vi "StartCore.vi"(8 "error in (no error)":errorcluster, 9 "Simulate?":bool, 10 "Service Details In":T1, 11 "MicronClient in":refnum<class "MicronClient.lvclass">) -> (0 "error out":errorcluster, 1 "Service Details Out":T1, 2 "Connection String":string, 3 "MicronClient out":refnum<class "MicronClient.lvclass">)   [LabVIEW 2019, in "MicronClient.lvclass"]
uses:
  MicronClient.lvclass
  Typedefs/ServiceDetails.ctl
  MicronCLI/Typedefs/Message.ctl
  MicronCLI/Typedefs/ServiceDetails.ctl
  824b107a-0fc2-4113-b1bd-0776a5adb667.vi
  <vilib>/SLL Toolkit/SLL String/_SubVIs/1D String Array to String.vi
  MicronCLI/MicronCLI.lvclass
  <vilib>/SLL Toolkit/SLL String/SLL String.lvlib
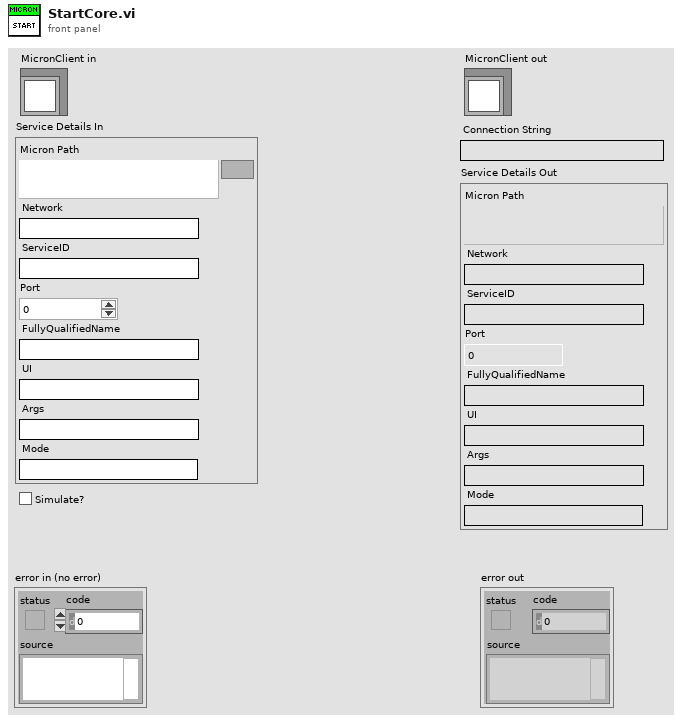
[diagram p1: front panel]
types:
  T1 = typedef "MicronClient.lvclass/ServiceDetails.ctl" = cluster{"Micron Path":path, "Network":string, "ServiceID":string, "Port":i32, "FullyQualifiedName":string, "UI":string, "Args":string, "Mode":string}
  T2 = typedef "MicronCLI.lvclass/Message.ctl" = cluster{"Command":string, "Payload":string}
  T3 = typedef "MicronCLI.lvclass/ServiceDetails.ctl" = cluster{"Network":string, "ServiceID":string}
  T4 = typedef "MicronClient.lvclass/MicronModeINISection.ctl" = cluster{"Command":string, "WorkingDirectory":path}
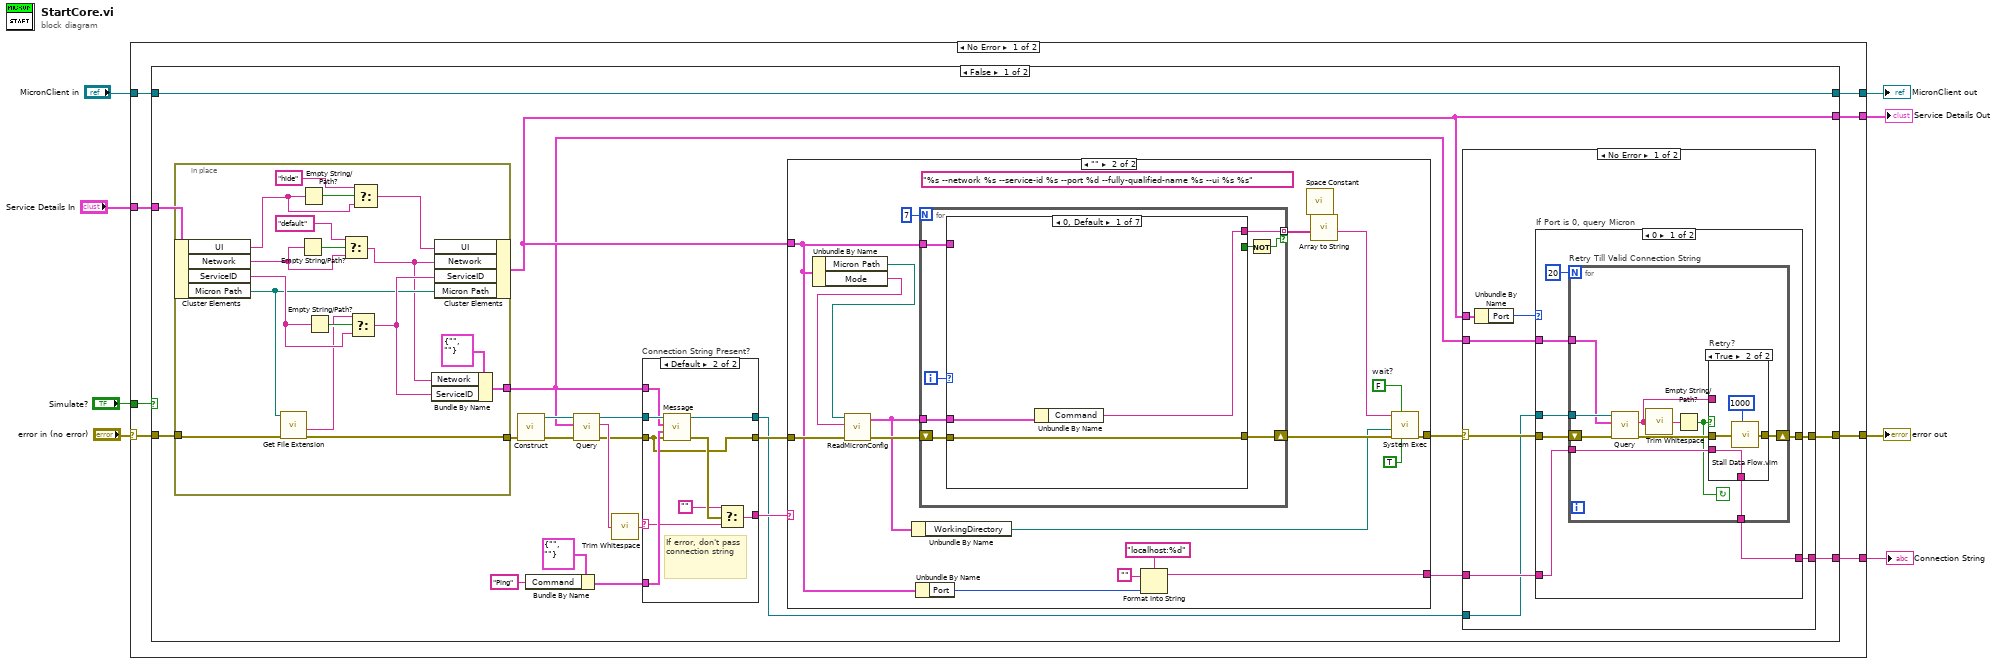
[diagram p0: block diagram]
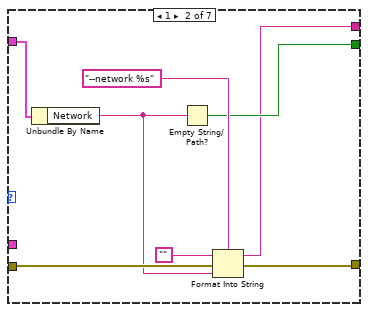
[diagram p7: hidden frame]
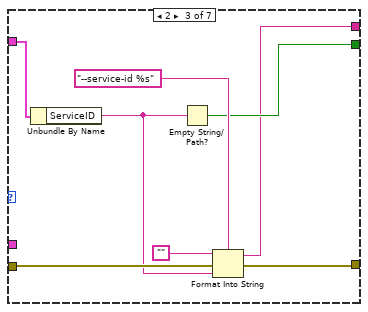
[diagram p8: hidden frame]
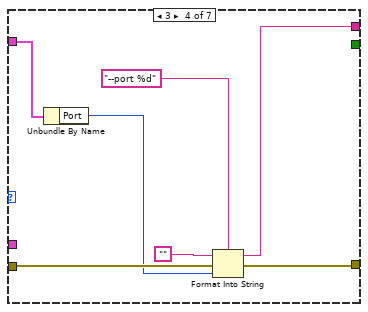
[diagram p9: hidden frame]
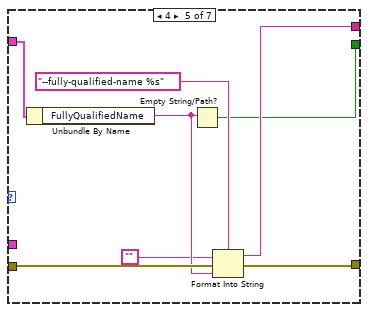
[diagram p10: hidden frame]
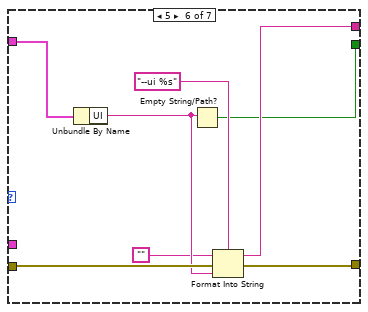
[diagram p11: hidden frame]
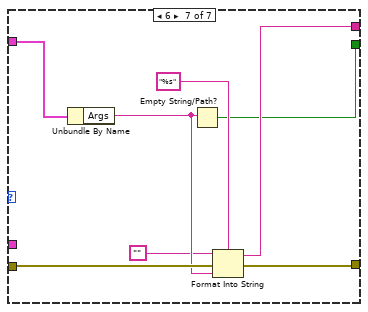
[diagram p12: hidden frame]
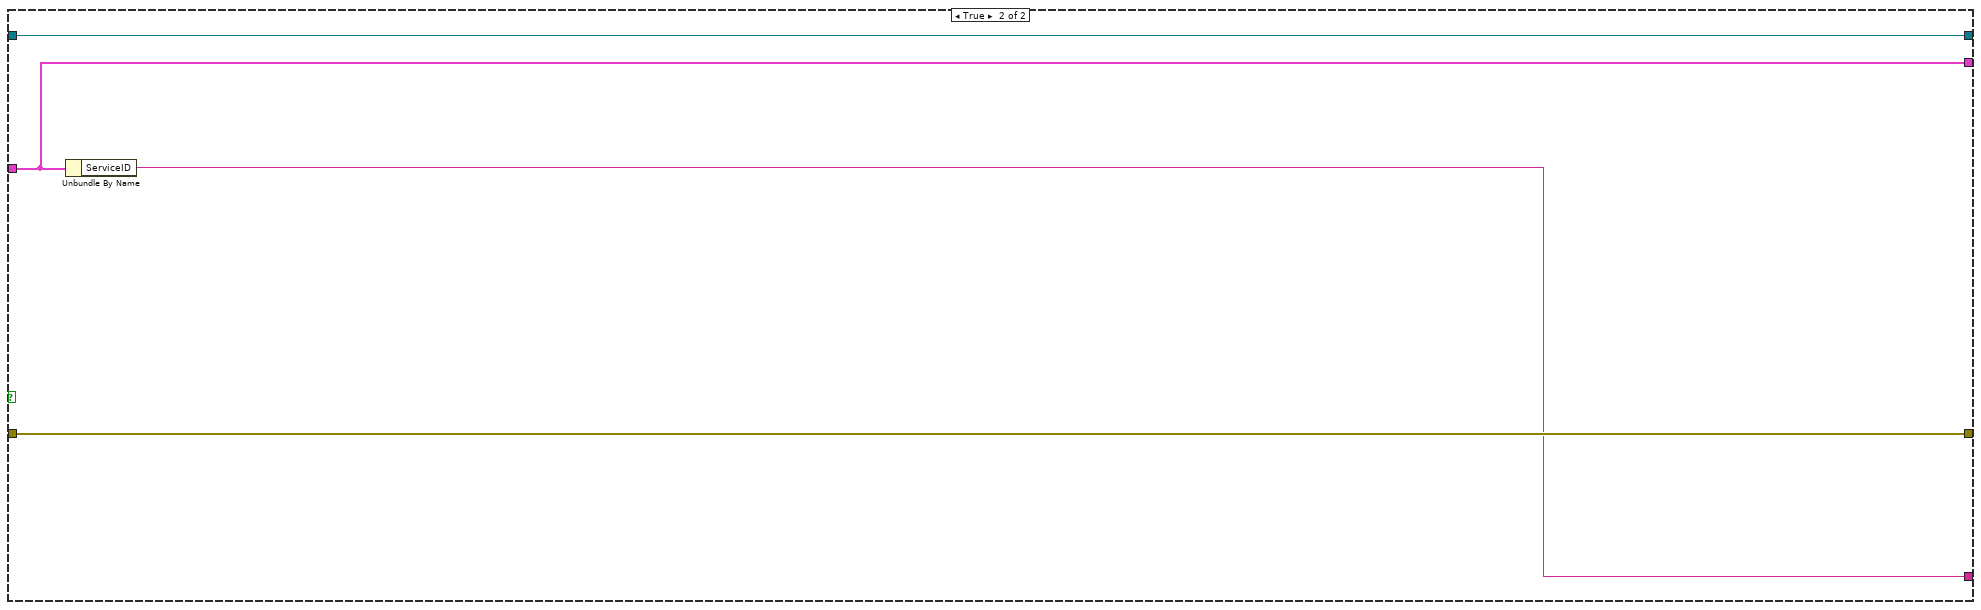
[diagram p13: hidden frame]
diagram:
  n1 = case shown="No Error" "error in (no error)" {
    selector: "error in (no error)" -> [w14 w188]
    tunnel: [w16 w188] -> w7
    tunnel: [w11 w187] -> w5
    tunnel: "MicronClient in" -> [w10 w187]
    tunnel: [w13 _] -> w4
    tunnel: "Service Details In" -> [w15 w186]
    tunnel: "Simulate?" -> [w12 _]
    tunnel: [w9 w186] -> w1
    frame No Error {
      n2 = case shown="False" w12 {
        tunnel: [w27 w185] -> w16
        tunnel: w15 -> [w38 w182]
        tunnel: w14 -> [w37 w185]
        tunnel: [w28 w183] -> w13
        tunnel: [w34 w184] -> w11
        tunnel: w10 -> [w34 w184]
        tunnel: [w30 w182] -> w9
        frame False {
          n3 = in-place {
            in-place-border: w37 -> [w178]
            in-place-border: [w174] -> w36
            in-place-border: [w165] -> w17
            n4 = in-place-cluster #1(w38) -> ("UI"=w170:string, "Network"=w180:string, "ServiceID"=w176:string, "Micron Path"=w173:path)
            n5 = call <vilib>:"Get File Extension.vi"("error in (no error)"=w178, "file"=w173) -> ("error out"=w174:errorcluster, "filename without extension"=w172:string)  [unwired: 5 in, 3 out]
            n6 = Empty String/Path?(string/path=w180) -> (empty?=w181:bool)
            n7 = Empty String/Path?(string/path=w170) -> (empty?=w171:bool)
            n8 = Empty String/Path?(string/path=w176) -> (empty?=w177:bool)
            n9 = Select(t="default", s=w181, f=w180) -> (s? t:f=w167:string)
            n10 = Select(t=w172, s=w177, f=w176) -> (s? t:f=w175:string)
            n11 = Select(t="hide", s=w171, f=w170) -> (s? t:f=w168:string)
            n12 = Bundle By Name(cluster=T3 {"Network"="", "ServiceID"=""} ("Service"), "Network"=w167, "ServiceID"=w175) -> (w165:T3)
            n13 = in-place-cluster #1("UI"=w168, "Network"=w167, "ServiceID"=w175, "Micron Path"=w173) -> (w30:T1)
          }
          n14 = call "Construct.vi"("error in (no error)"=w36) -> ("error out"=w33:errorcluster, "MicronCLI out"=w32:refnum<class "MicronCLI.lvclass">)  [unwired: 9 in]
          n15 = Bundle By Name(cluster=T2 {"Command"="", "Payload"=""} ("Message"), "Command"="Ping") -> (w18:T2)
          n16 = call-dynamic "Query.vi"("error in (no error)"=w33, "Service"=w17, "MicronCLI in"=w32) -> ("error out"=w26:errorcluster, "ConnectionString"=w35:string, "MicronCLI out"=w25:refnum<class "MicronCLI.lvclass">)  [unwired: 6 in]
          n17 = call <vilib>:"Trim Whitespace.vi"("string"=w35) -> ("trimmed string"=w24:string)  [unwired: 1 in]
          n18 = case "Connection String Present?" shown="Default" w24 {
            selector: w24 -> [w75 w79]
            tunnel: w26 -> [w76 w77]
            tunnel: w25 -> [w74 w85]
            tunnel: w17 -> [_ w84]
            tunnel: [w76 w77] -> w23
            tunnel: [w75 w78] -> w22
            tunnel: [w74 w83] -> w21
            tunnel: w18 -> [_ w82]
            frame "" {
            }
            frame Default {
              # "If error, don't pass connection string"
              n19 = call-dynamic "Message.vi"("error in (no error)"=w77, "Message"=w82, "Service"=w84, "MicronCLI in"=w85) -> ("error out"=w81:errorcluster, "MicronCLI out"=w83:refnum<class "MicronCLI.lvclass">)  [unwired: 5 in, 1 out]
              n20 = Select(t="", s=w81, f=w79) -> (s? t:f=w78:string)
            }
          }
          n21 = case shown="\"\"" w22 {
            selector: w22 -> [w87 _]
            tunnel: [w86 w98] -> w29
            tunnel: w30 -> [_ w92]
            tunnel: [w87 w96] -> w31
            tunnel: w23 -> [w86 w94]
            frame Default {
            }
            frame "" {
              (unwired) "%s --network %s --service-id %s --port %d --fully-qualified-name %s --ui %s %s" ("format string")
              w106 = FALSE  # wait?
              n22 = Unbundle By Name(w92) -> ("Micron Path"=w91:path, "Mode"=w88:string)
              n23 = call "ReadMicronConfig.vi"("Error In"=w94, "Mode"=w88, "Micron Path In"=w91) -> ("Error Out"=w93:errorcluster, "Micron Mode"=w90:T4)  [unwired: 7 in]
              n24 = Unbundle By Name(w90) -> ("WorkingDirectory"=w89:path)
              n25 = Unbundle By Name(w92) -> ("Port"=w97:i32)
              n26 = for {
                N: 7 -> [_]
                tunnel: w92 -> [w113]
                shift-right: [w111] -> w105
                shift-left: w93 -> [w112]
                tunnel: [w110] -> w101 mode=indexing if=w108
                tunnel: w90 -> [w107]
                i -> [w114]
                n27 = case shown="0, Default" w114 {
                  tunnel: w113 -> [_ w125 w133 w140 w148 w156 w164]
                  tunnel: w112 -> [w115 w124 w132 w139 w147 w155 w163]
                  tunnel: [w115 w123 w131 w138 w146 w154 w162] -> w111
                  tunnel: [w117 w119 w127 w135 w144 w152 w160] -> w110
                  tunnel: [_ w120 w128 _ w142 w150 w158] -> w109
                  tunnel: w107 -> [w116 _ _ _ _ _ _]
                  frame 0, Default {
                    n28 = Unbundle By Name(w116) -> ("Command"=w117:string)
                  }
                  frame 1 {
                    n29 = Unbundle By Name(w125) -> ("Network"=w121:string)
                    n30 = Empty String/Path?(string/path=w121) -> (empty?=w120:bool)
                    n31 = Format Into String(format string="--network %s", initial string="", error in=w124, w121) -> (resulting string=w119:string, error out=w123:errorcluster)
                  }
                  frame 2 {
                    n32 = Unbundle By Name(w133) -> ("ServiceID"=w129:string)
                    n33 = Empty String/Path?(string/path=w129) -> (empty?=w128:bool)
                    n34 = Format Into String(format string="--service-id %s", initial string="", error in=w132, w129) -> (resulting string=w127:string, error out=w131:errorcluster)
                  }
                  frame 3 {
                    n35 = Unbundle By Name(w140) -> ("Port"=w136:i32)
                    n36 = Format Into String(format string="--port %d", initial string="", error in=w139, w136) -> (resulting string=w135:string, error out=w138:errorcluster)
                  }
                  frame 4 {
                    n37 = Unbundle By Name(w148) -> ("FullyQualifiedName"=w143:string)
                    n38 = Empty String/Path?(string/path=w143) -> (empty?=w142:bool)
                    n39 = Format Into String(format string="--fully-qualified-name %s", initial string="", error in=w147, w143) -> (resulting string=w144:string, error out=w146:errorcluster)
                  }
                  frame 5 {
                    n40 = Unbundle By Name(w156) -> ("UI"=w151:string)
                    n41 = Empty String/Path?(string/path=w151) -> (empty?=w150:bool)
                    n42 = Format Into String(format string="--ui %s", initial string="", error in=w155, w151) -> (resulting string=w152:string, error out=w154:errorcluster)
                  }
                  frame 6 {
                    n43 = Unbundle By Name(w164) -> ("Args"=w159:string)
                    n44 = Empty String/Path?(string/path=w159) -> (empty?=w158:bool)
                    n45 = Format Into String(format string="%s", initial string="", error in=w163, w159) -> (resulting string=w160:string, error out=w162:errorcluster)
                  }
                }
                n46 = Not(x=w109) -> (.not. x?=w108:bool)
              }
              n47 = Format Into String(format string="localhost:%d", initial string="", w97) -> (resulting string=w96:string)  [unwired: 1 in, 1 out]
              n48 = call <vilib>:"Space Constant.vi"() -> ("String"=w100:string)
              n49 = call-poly <vilib>:"Array to String.vi"("Delimiter (,)"=w100, "1D Array[]"=w101) -> ("String"=w104:string)  [unwired: 6 in]
              n50 = call <vilib>:"System Exec.vi"("run minimized? (F)"=TRUE, "wait until completion? (T)"=w106, "error in (no error)"=w105, "working directory"=w89, "command line"=w104) -> ("error out"=w98:errorcluster)  [unwired: 3 in, 3 out]
            }
          }
          n51 = case shown="No Error" w29 {
            selector: w29 -> [w43 w73]
            tunnel: w31 -> [w46 w72]
            tunnel: w30 -> [w45 _]
            tunnel: [w42 w72] -> w28
            tunnel: [w41 w73] -> w27
            tunnel: w21 -> [w40 _]
            tunnel: w17 -> [w39 _]
            frame No Error {
              n52 = Unbundle By Name(w45) -> ("Port"=w44:i32)
              n53 = case "If Port is 0, query Micron" shown="0" w44 {
                tunnel: w46 -> [w48 w71]
                tunnel: w43 -> [w53 w70]
                tunnel: [w49 w71] -> w42
                tunnel: [w52 w70] -> w41
                tunnel: w40 -> [w51 _]
                tunnel: w39 -> [w47 _]
                frame 0 {
                  n54 = for "Retry Till Valid Connection String" {
                    N: 20 -> [_]
                    tunnel: w51 -> [w62]
                    shift-right: [w60] -> w52
                    shift-left: w53 -> [w63]
                    tunnel: [w59] -> w49
                    tunnel: w48 -> [w58]
                    tunnel: w47 -> [w54]
                    stop <- w55 continue-if-true
                    n55 = call-dynamic "Query.vi"("error in (no error)"=w63, "Service"=w54, "MicronCLI in"=w62) -> ("error out"=w61:errorcluster, "ConnectionString"=w56:string)  [unwired: 6 in, 1 out]
                    n56 = call <vilib>:"Trim Whitespace.vi"("string"=w56) -> ("trimmed string"=w57:string)  [unwired: 1 in]
                    n57 = Empty String/Path?(string/path=w57) -> (empty?=w55:bool)
                    n58 = case "Retry?" shown="True" w55 {
                      tunnel: w61 -> [w65 w69]
                      tunnel: [w65 w68] -> w60
                      tunnel: [w64 w67] -> w59
                      tunnel: w58 -> [_ w67]
                      tunnel: w56 -> [w64 _]
                      frame False {
                      }
                      frame True {
                        n59 = call "Stall Data Flow.vim"("value in"=w69, "milliseconds to wait"=u32 1000) -> ("value out"=w68:errorcluster)  [unwired: 1 out]
                      }
                    }
                  }
                }
                frame 1, Default {
                }
              }
            }
            frame Error {
            }
          }
        }
        frame True {
          n60 = Unbundle By Name(w182) -> ("ServiceID"=w183:string)
        }
      }
    }
    frame Error {
    }
  }
  "error out" <- w7
  "MicronClient out" <- w5
  "Connection String" <- w4
  "Service Details Out" <- w1
